vi "scale sliders Write.vi"(4 "error in (no error)":errorcluster, 5 "Value":bool, 6 "Container State":T2, 7 "Display State In":T1={"X cursor"={"state"=enum."cursor and slider", "color"=6618880}, "Y cursor"={"state"=enum."cursor and slider", "color"=6618880}, "Scale Sliders"=FALSE}) -> (0 "error out":errorcluster, 3 "Display State Out":T1={"X cursor"={"state"=enum."cursor and slider", "color"=6618880}, "Y cursor"={"state"=enum."cursor and slider", "color"=6618880}, "Scale Sliders"=FALSE})   [LabVIEW 2016, in "CursorImageControl.xctl"]
uses:
  CursorImageControl.xctl
  <vilib>/_xctls/Container State.ctl
  State.ctl
  <vilib>/_xctls/XControlSupport.lvlib
panel:
  # "Replace the Value Control below with a Control of desired type.\nDo not remove this Control or the others from the connector pane.\nDo not change the connector pane pattern.\nThe Value control should always be the third terminal from top on the input side in the connector pane."
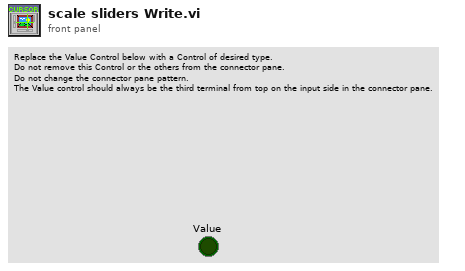
[diagram p1: front panel]
types:
  T1 = typedef "CursorImageControl.xctl/State.ctl" = cluster{"X cursor":cluster{"state":enum16{"cursor and slider", "cursor only", "hide all"}, "color":u32}, "Y cursor":cluster{"state":enum16{"cursor and slider", "cursor only", "hide all"}, "color":u32}, "Scale Sliders":bool}
  T2 = typedef "XControlSupport.lvlib/Container State.ctl" = cluster{"Indicator?":bool, "Run Mode?":bool, " Refnum":refnum<vi>}
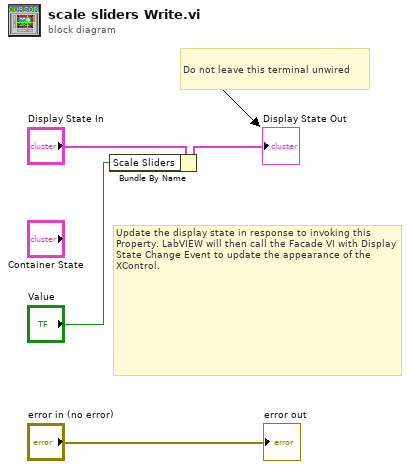
[diagram p0: block diagram]
diagram:
  # "Do not leave this terminal unwired"
  # "Update the display state in response to invoking this Property. LabVIEW will then call the Facade VI with Display State Change Event to update the appearance of the XControl."
  n1 = Bundle By Name(cluster="Display State In", "Scale Sliders"="Value") -> (→"Display State Out":T1)
  "error out" <- "error in (no error)"
